vi "Read Bytes.vi"(8 "error in (no error)":errorcluster, 10 "Bytes to Read":i32, 11 "ProtectedConnectionReader":refnum<class "ProtectedConnectionReader.lvclass">) -> (0 "error out":errorcluster, 3 "Message":string)   [LabVIEW 2019, in "Network Messenger.lvlib" / "ReadStrategy.lvclass"]
uses:
  <vilib>/gpm_packages/@cs/Network-interface/Source/Network Messenger/ReadStrategy/ReadStrategy.lvclass
  <vilib>/gpm_packages/@cs/Network-interface/Source/ProtectedConnectionReader/ProtectedConnectionReader.lvclass
  <vilib>/gpm_packages/@cs/Network-interface/Source/ProtectedConnectionReader/ProtectedConnectionReader.lvclass/ProtectedConnectionReader.ctl
  <vilib>/gpm_packages/@cs/Network-interface/Source/Connection Reference/Connection Reference/Connection Reference.lvclass/Connection Reference.ctl
  <vilib>/Utility/error.llb/Error Cluster From Error Code.vi
  <vilib>/gpm_packages/@cs/Network-interface/Source/Connection Reference/IConnection/IConnection.lvclass
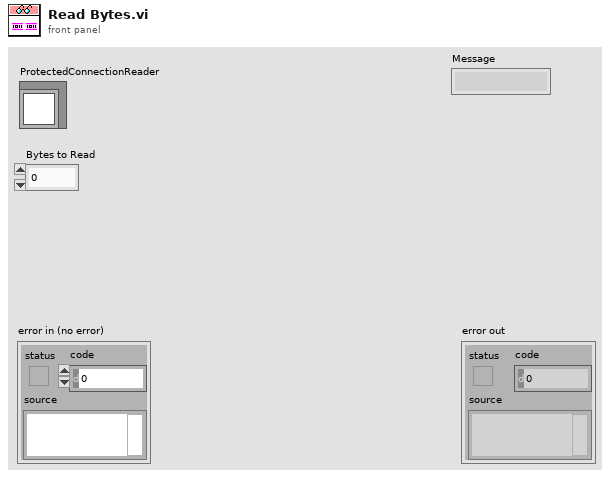
[diagram p1: front panel]
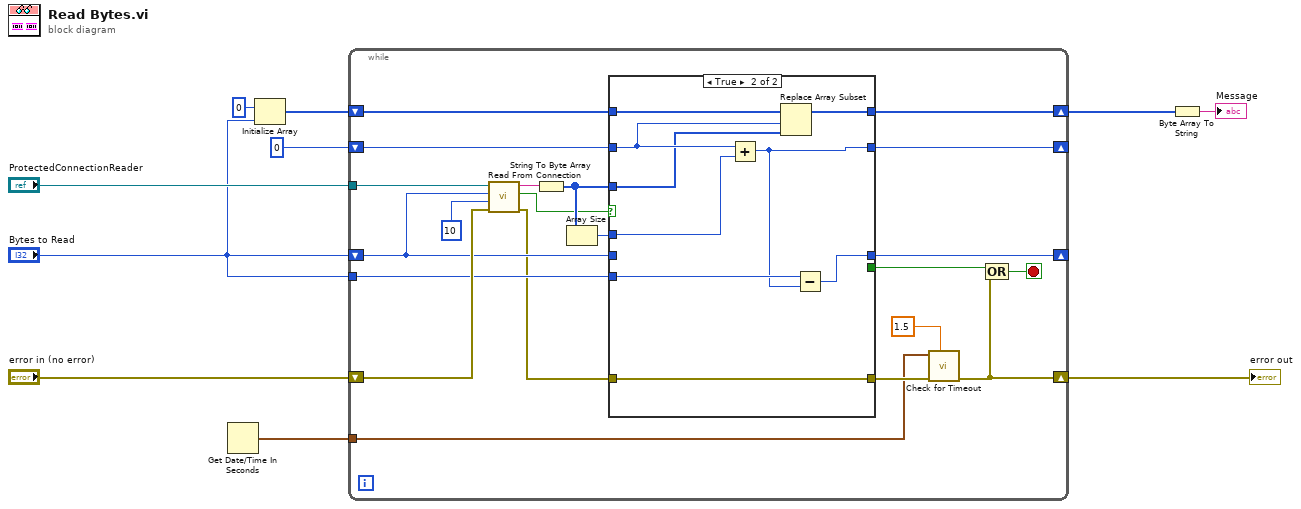
[diagram p0: block diagram]
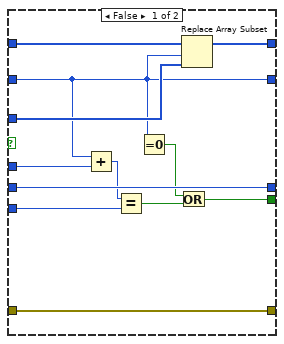
[diagram p2: hidden frame]
diagram:
  n1 = Get Date/Time In Seconds() -> (seconds since 1Jan1904=w2:timestamp)
  n2 = Initialize Array(u8 0 ("element"), "Bytes to Read") -> (w6:u8[])
  n3 = while {
    tunnel: "ProtectedConnectionReader" -> [w31]
    shift-right: [w14] -> w8
    shift-left: "error in (no error)" -> [w29]
    shift-right: [w26] -> w4
    shift-left: w6 -> [w28]
    shift-right: [w25] -> _
    shift-left: 0 -> [w27]
    tunnel: w2 -> [w12]
    shift-right: [w21] -> _
    shift-left: "Bytes to Read" -> [w24]
    tunnel: "Bytes to Read" -> [w17]
    stop <- w19 stop-if-true
    n4 = call <vilib>:"Read From Connection.vi"("error in (no error)"=w29, "Timeout (ms)"=10, "Bytes to Read"=w24, "ProtectedConnectionReader in"=w31) -> ("error out"=w15:errorcluster, "TimeOut?"=w20:bool, "Data"=w23:string)  [unwired: 5 in]
    n5 = String To Byte Array(string=w23) -> (unsigned byte array=w22:u8[])
    n6 = Array Size(array=w22) -> (size(s)=w16:i32)
    n7 = case shown="True" w20 {
      tunnel: w28 -> [w41 w50]
      tunnel: w27 -> [w37 w49]
      tunnel: [w42 w51] -> w26
      tunnel: [w37 w45] -> w25
      tunnel: w24 -> [w43 _]
      tunnel: w22 -> [w39 w48]
      tunnel: [w43 w44] -> w21
      tunnel: [w34 _] -> w18
      tunnel: w17 -> [w40 w46]
      tunnel: w16 -> [w33 w47]
      tunnel: w15 -> [w32 w52]
      tunnel: [w32 w52] -> w13
      frame False {
        n8 = Add(x=w37, y=w33) -> (x+y=w38:i32)
        n9 = Equal?(x=w38, y=w40) -> (x = y?=w36:bool)
        n10 = Equal To 0?(x=w37) -> (x = 0?=w35:bool)
        n11 = Or(x=w35, y=w36) -> (x .or. y?=w34:bool)
        n12 = Replace Array Subset(array=w41, new element=w39, index=w37) -> (w42:u8[])
      }
      frame True {
        n13 = Add(x=w49, y=w47) -> (x+y=w45:i32)
        n14 = Replace Array Subset(array=w50, new element=w48, index=w49) -> (w51:u8[])
        n15 = Subtract(x=w46, y=w45) -> (x-y=w44:i32)
      }
    }
    n16 = call <vilib>:"Check for Timeout.vi"("Timeout(S)"=1.5, "error in (no error)"=w13, "Start Time"=w12) -> ("error out"=w14:errorcluster)  [unwired: 8 in]
    n17 = Compound Arithmetic op=OR(w18, w14) -> (w19:bool)
  }
  "error out" <- w8
  n18 = Byte Array To String(unsigned byte array=w4) -> (string=→"Message":string)
